vi "Create Placeholder Channel Names.vi"(10 "Count":i32, 11 "Group Name":string) -> (3 "Channels":T1[](array[typedef]))   [LabVIEW 2020, in "Vecto.lvlib" / "RemoteDataService.lvclass"]
uses:
  RemoteDataService.lvclass
  RemoteDataService.lvclass/RemoteDataService.ctl
  Channel Init.ctl
  Vecto.lvlib
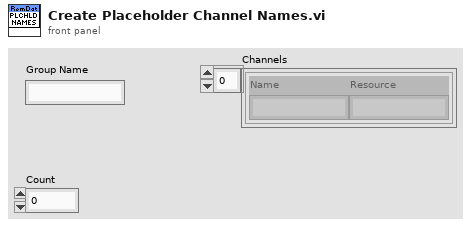
[diagram p1: front panel]
types:
  T1 = typedef "Vecto.lvlib/Channel Init.ctl" = cluster{"Name":string, "Resource":string}
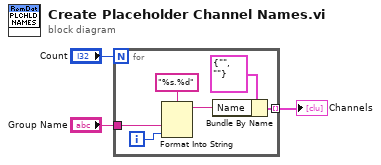
[diagram p0: block diagram]
diagram:
  n1 = for {
    N: "Count" -> [_]
    tunnel: "Group Name" -> [w8]
    tunnel: [w4] -> w1 mode=indexing
    i -> [w7]
    n2 = Format Into String(format string="%s.%d", w8, w7) -> (resulting string=w5:string)  [unwired: 2 in, 1 out]
    n3 = Bundle By Name(cluster=T1 {"Name"="", "Resource"=""} ("Channel Init"), "Name"=w5) -> (w4:T1)
  }
  "Channels" <- w1
